vi "PathVelocityProfile.vi"(0 "Pose":dbl[](array[numeric]), 1 "time":dbl, 3 "intervalo":dbl=0.016, 5 "estimatives":T2, 9 "Path  Smooth":dbl[][](array[numeric]), 11 "V_max":dbl format="%#_13g", 13 "Accel":dbl=10.0, 14 "DesAccel":dbl=15.0) -> (4 "Time X":dbl[](array[numeric]), 6 "Velocities X":dbl[](array[numeric]), 8 "Time Y":dbl[](array[numeric]), 10 "Velocities Y":dbl[](array[numeric]))   [LabVIEW 2023]
uses:
  Controle/VelocityProfileState.ctl
  <vilib>/Analysis/_algsub.llb/Real Vector Norm.vi
  <vilib>/Analysis/coordinate.llb/Wrap Angle (scalar).vi
  <vilib>/Analysis/NI_AAL_Angle.lvlib
  <vilib>/Analysis/NI_AALPro.lvlib
panel:
  in  "est_vy":dbl
  in  "est_vx":dbl
  out "VelocityProfile Y":T1[](array[typedef])
  out "VelocityProfile X":T1[](array[typedef])
  out "Velocity Profile Y":cluster{dbl[], dbl[]}[](graph)
  out "Velocity Profile X":cluster{dbl[], dbl[]}[](graph)
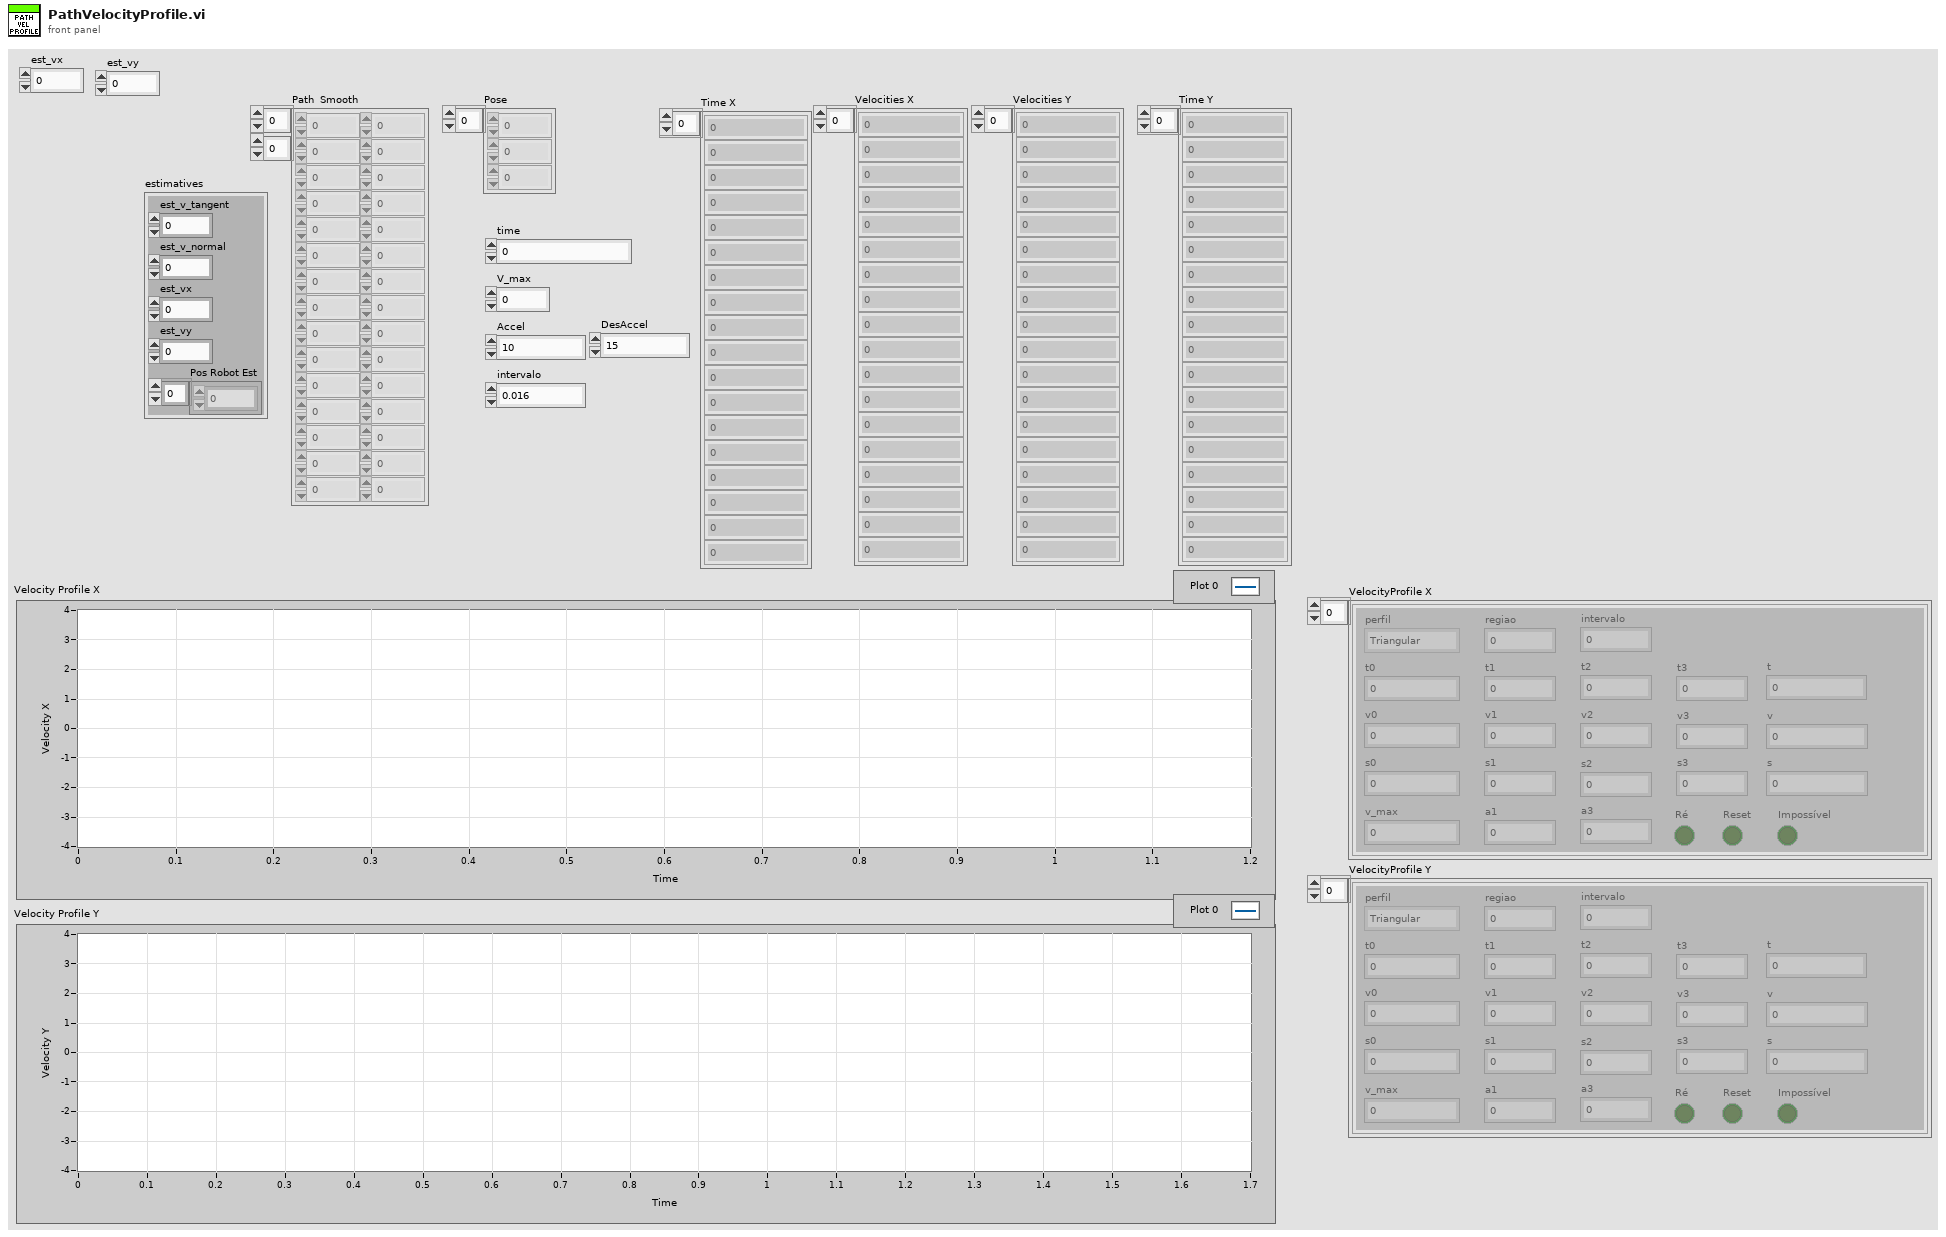
[diagram p1: front panel]
types:
  T1 = typedef "VelocityProfileState.ctl" = cluster{"t0":dbl, "t1":dbl, "t2":dbl, "t3":dbl, "v0":dbl, "v_max":dbl, "v3":dbl, "v2":dbl, "v1":dbl, "perfil":enum16{"Triangular", "Trapezoidal"}, "regiao":i32, "s0":dbl, "s1":dbl, "s2":dbl, "v":dbl, "t":dbl, "a1":dbl, "s3":dbl, "Reset":bool, "s":dbl, "a3":dbl, "Ré":bool, "Impossível":bool, "intervalo":dbl}
  T2 = cluster{"est_v_tangent":dbl, "est_v_normal":dbl, "est_vx":dbl, "est_vy":dbl, "Pos Robot Est":dbl[]}
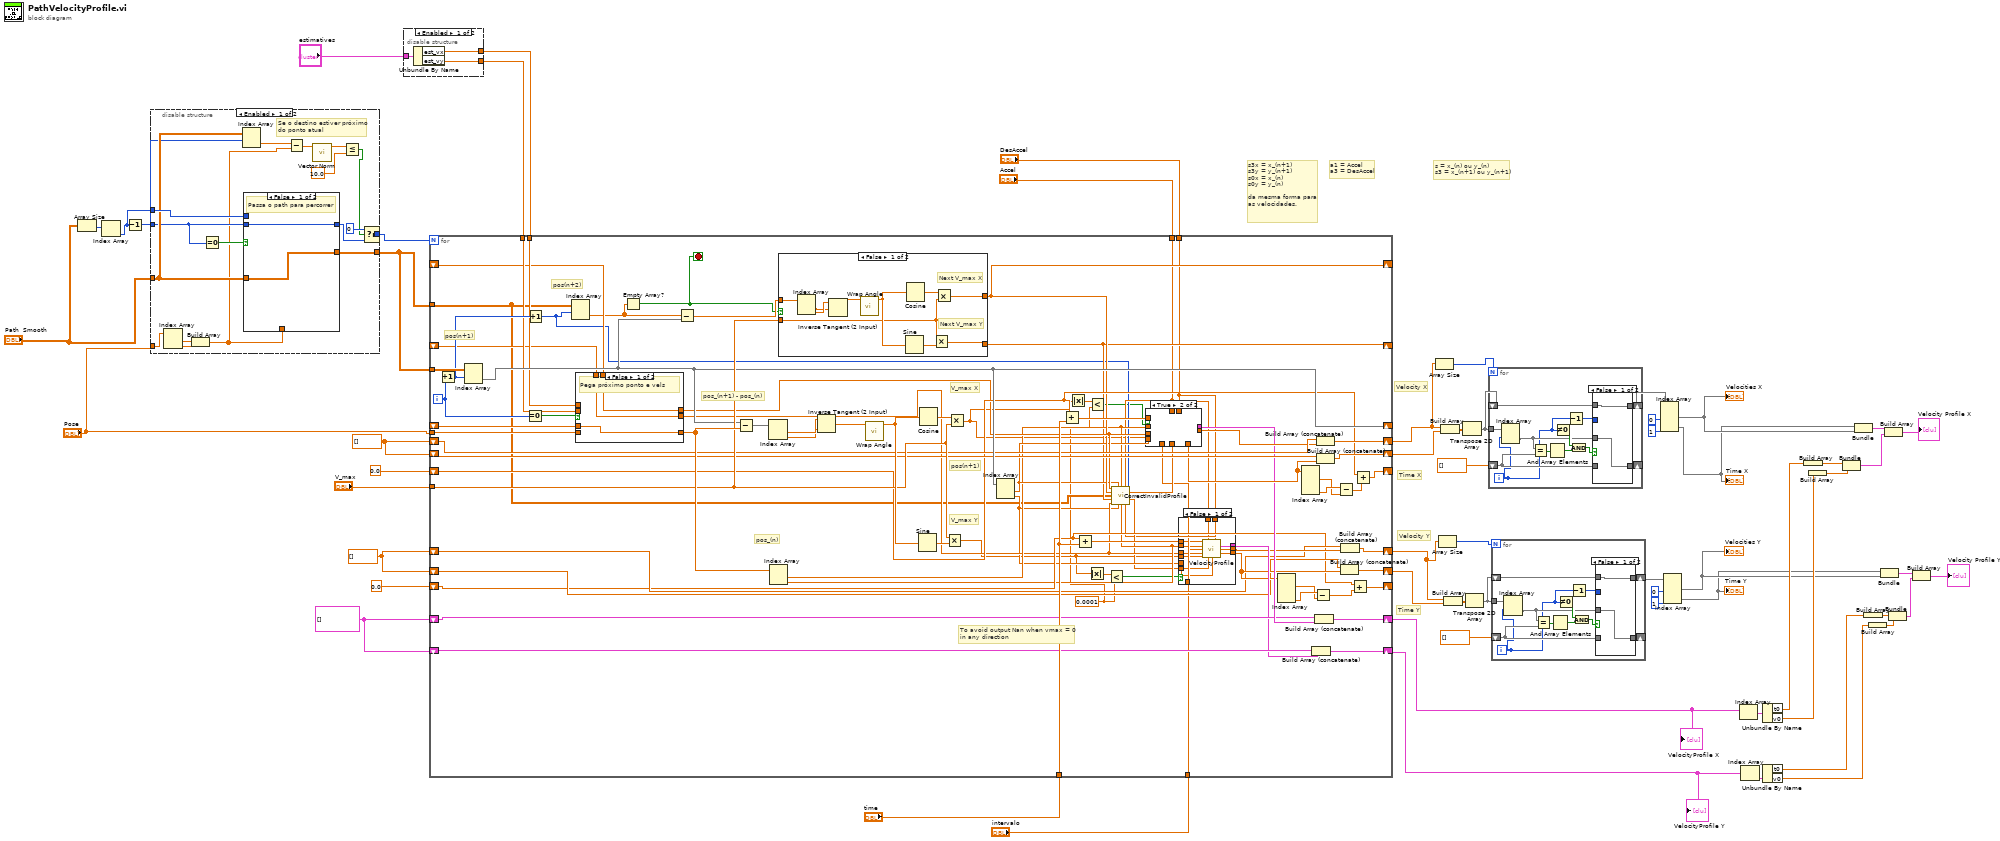
[diagram p0: block diagram]
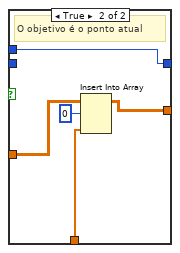
[diagram p2: hidden frame]
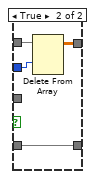
[diagram p4: hidden frame]
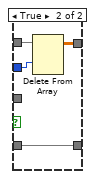
[diagram p5: hidden frame]
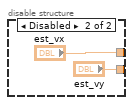
[diagram p6: hidden frame]
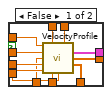
[diagram p7: hidden frame]
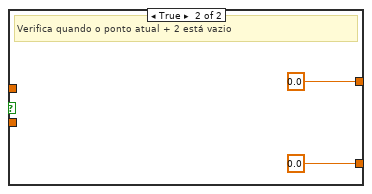
[diagram p9: hidden frame]
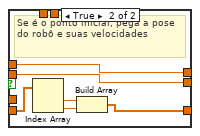
[diagram p10: hidden frame]
diagram:
  w48 = T1[] []
  w50 = dbl[] []
  w49 = dbl[] []
  # "s = x_(n) ou y_(n)\ns3 = x_(n+1) ou y_(n+1)"
  # "a1 = Accel\na3 = DesAccel"
  # "s3x = x_(n+1)\ns3y = y_(n+1)\ns0x = x_(n)\ns0y = y_(n)\n\nda mesma forma para\nas velocidades."
  # "Time X"
  # "Time Y"
  # "Velocity Y"
  # "Velocity X"
  n1 = Array Size(array="Path  Smooth") -> (size(s)=w53:i32[])
  n2 = Index Array(array=w53) -> (element=w6:i32)  [unwired: 1 in]
  n3 = Decrement(x=w6) -> (x-1=w3:i32)
  n4 = disable-structure shown="Enabled" {
    disable-tunnel: [w77 w85] -> w2
    disable-tunnel: w6 -> [w75 _]
    disable-tunnel: "Pose" -> [w74 _]
    disable-tunnel: [w71 w86] -> w1
    disable-tunnel: "Path  Smooth" -> [w68 w85]
    disable-tunnel: w3 -> [w67 w86]
    frame Enabled {
      # "Se o destino estiver próximo\ndo ponto atual"
      n5 = Index Array(array=w74) -> (element #1=w73:dbl, element #2=w72:dbl)  [unwired: 2 in]
      n6 = Build Array(w73, w72) -> (w65:dbl[])
      n7 = Equal To 0?(x=w67) -> (x = 0?=w76:bool)
      n8 = Index Array(array=w68, index (row)=w67) -> (element=w66:dbl[])  [unwired: 1 in]
      n9 = case shown="False" w76 {
        tunnel: [w78 w80] -> w77
        tunnel: w68 -> [w78 w82]
        tunnel: [w79 w84] -> w70
        tunnel: w67 -> [w79 _]
        tunnel: w75 -> [_ w84]
        tunnel: w65 -> [_ w83]
        frame False {
          # "Passa o path para percorrer"
        }
        frame True {
          # "O objetivo é o ponto atual"
          n10 = Insert Into Array(array=w82, index (row)=0, new element=w83) -> (w80:dbl[][])  [unwired: 1 in]
        }
      }
      n11 = Subtract(x=w66, y=w65) -> (x-y=w64:dbl[])
      n12 = call-poly <vilib>:"Vector Norm.vi"("Input Vector"=w64) -> ("norm"=w63:dbl)  [unwired: 9 in, 1 out]
      n13 = Less Or Equal?(x=w63, y=10.0) -> (x <= y?=w61:bool)
      n14 = Select(t=0, s=w61, f=w70) -> (s? t:f=w71:i32)
    }
    frame Disabled {
    }
  }
  n15 = disable-structure shown="Enabled" {
    disable-tunnel: "estimatives" -> [w89 _]
    disable-tunnel: [w88 "est_vx"] -> w52
    disable-tunnel: [w87 "est_vy"] -> w51
    frame Enabled {
      n16 = Unbundle By Name(w89) -> ("est_vx"=w88:dbl, "est_vy"=w87:dbl)
    }
    frame Disabled {
    }
  }
  n17 = for {
    N: w1 -> [_]
    tunnel: w2 -> [w150]
    tunnel: "Pose" -> [w166]
    shift-right: [w151] -> _
    shift-left: _ -> [w165]
    tunnel: "V_max" -> [w155]
    tunnel: "Accel" -> [w105]
    tunnel: "DesAccel" -> [w104]
    tunnel: w2 -> [w101]
    shift-right: [w119] -> _
    shift-left: 0.0 ("t3") -> [w121]
    shift-right: [w117] -> _
    shift-left: 0.0 ("t3") -> [w116]
    tunnel: "time" -> [w153]
    shift-right: [w144] -> w27
    shift-left: w49 -> [w149]
    shift-right: [w147] -> w30
    shift-left: w49 -> [w148]
    shift-right: [w125] -> w9
    shift-left: w50 -> [w123]
    shift-right: [w124] -> w10
    shift-left: w50 -> [w122]
    tunnel: w52 -> [w141]
    tunnel: w51 -> [w140]
    shift-right: [w114] -> _
    shift-left: _ -> [w139]
    shift-right: [w108] -> _
    shift-left: _ -> [w138]
    shift-right: [w130] -> w46
    shift-left: w48 -> [w133]
    shift-right: [w129] -> w45
    shift-left: w48 -> [w132]
    tunnel: "intervalo" -> [w99]
    i -> [w102]
    stop <- w142 stop-if-true
    w93 = 0.0001 ("y")
    # "To avoid output Nan when vmax = 0\nin any direction"
    # "pos(n+2)"
    # "pos(n+1)"
    # "pos(n+1)"
    # "pos_(n)"
    # "pos_(n+1) - pos_(n)"
    # "V_max Y"
    # "V_max X"
    n18 = Increment(x=w102) -> (x+1=w146:i32)
    n19 = Index Array(array=w150, index (row)=w146) -> (element=w151:dbl[])  [unwired: 1 in]
    n20 = Equal To 0?(x=w102) -> (x = 0?=w167:bool)
    n21 = Increment(x=w146) -> (x+1=w100:i32)
    n22 = Index Array(array=w101, index (row)=w100) -> (element=w103:dbl[])  [unwired: 1 in]
    n23 = case shown="False" w167 {
      tunnel: w166 -> [_ w212]
      tunnel: [w206 w209] -> w157
      tunnel: w165 -> [w206 _]
      tunnel: w141 -> [_ w208]
      tunnel: w140 -> [_ w207]
      tunnel: [w204 w208] -> w115
      tunnel: [w205 w207] -> w110
      tunnel: w139 -> [w204 _]
      tunnel: w138 -> [w205 _]
      frame False {
        # "Pega próximo ponto e vels"
      }
      frame True {
        # "Se é o ponto inicial, pega a pose\ndo robô e suas velocidades"
        n24 = Index Array(array=w212) -> (element #1=w211:dbl, element #2=w210:dbl)  [unwired: 2 in]
        n25 = Build Array(w211, w210) -> (w209:dbl[])
      }
    }
    n26 = Empty Array?(array=w103) -> (empty?=w142:bool)
    n27 = Subtract(x=w103, y=w151) -> (x-y=w156:dbl[])
    n28 = Subtract(x=w151, y=w157) -> (x-y=w163:dbl[])
    n29 = Index Array(array=w163) -> (element #1=w164:dbl, element #2=w162:dbl)  [unwired: 2 in]
    n30 = Index Array(array=w157) -> (element #1=w112:dbl, element #2=w111:dbl)  [unwired: 2 in]
    n31 = case shown="False" w142 {
      tunnel: w156 -> [w196 _]
      tunnel: w155 -> [w194 _]
      tunnel: [w193 0.0] -> w114
      tunnel: [w192 0.0] -> w108
      frame False {
        # "Next V_max Y"
        # "Next V_max X"
        n32 = Index Array(array=w196) -> (element #1=w195:dbl, element #2=w197:dbl)  [unwired: 2 in]
        n33 = Inverse Tangent (2 Input)(1:w195, 2:w197) -> (0:w198:dbl)
        n34 = call-poly <vilib>:"Wrap Angle.vi"("angle in"=w198) -> ("angle out"=w199:dbl)  [unwired: 9 in, 1 out]
        n35 = Sine(x=w199) -> (sin(x)=w201:dbl)
        n36 = Cosine(x=w199) -> (cos(x)=w200:dbl)
        n37 = Multiply(x=w194, y=w201) -> (x*y=w192:dbl)
        n38 = Multiply(x=w200, y=w194) -> (x*y=w193:dbl)
      }
      frame True {
        # "Verifica quando o ponto atual + 2 está vazio"
      }
    }
    n39 = Inverse Tangent (2 Input)(1:w164, 2:w162) -> (0:w161:dbl)
    n40 = call-poly <vilib>:"Wrap Angle.vi"("angle in"=w161) -> ("angle out"=w160:dbl)  [unwired: 9 in, 1 out]
    n41 = Sine(x=w160) -> (sin(x)=w158:dbl)
    n42 = Cosine(x=w160) -> (cos(x)=w159:dbl)
    n43 = Multiply(x=w155, y=w158) -> (x*y=w98:dbl)
    n44 = Multiply(x=w159, y=w155) -> (x*y=w94:dbl)
    n45 = Index Array(array=w151) -> (element #1=w113:dbl, element #2=w109:dbl)  [unwired: 2 in]
    n46 = Add(x=w121, y=w153) -> (x+y=w154:dbl)
    n47 = Absolute Value(x=w94) -> (abs(x)=w95:dbl)
    n48 = Add(x=w116, y=w153) -> (x+y=w152:dbl)
    n49 = Absolute Value(x=w98) -> (abs(x)=w97:dbl)
    n50 = Less?(x=w95, y=w93) -> (x < y?=w92:bool)
    n51 = Less?(x=w97, y=w93) -> (x < y?=w96:bool)
    n52 = call "CorrectInvalidProfile.vi"("v0x"=w115, "s3x"=w113, "s0x"=w112, "a1"=w105, "index"=w100, "v3x"=w114, "Path  Smooth"=w101, "v3y"=w108, "v0y"=w110, "s3y"=w109, "s0y"=w111, "a3"=w104) -> ("New v3x"=w106:dbl, "New v3y"=w107:dbl)  [unwired: 2 in]
    n53 = case shown="True" w92 {
      tunnel: w94 -> [w179 _]
      tunnel: w154 -> [w178 _]
      tunnel: [w177 _] -> w145
      tunnel: [w176 _] -> w143
      tunnel: [w175 _] -> w134
      tunnel: w115 -> [w174 _]
      tunnel: w113 -> [w173 _]
      tunnel: w112 -> [w172 _]
      tunnel: w106 -> [w171 _]
      tunnel: w105 -> [w170 _]
      tunnel: w104 -> [w169 _]
      tunnel: w99 -> [w168 _]
      frame False {
        n54 = call "VelocityProfile.vi"("t"=w178, "a1"=w170, "a3"=w169, "s"=w172, "intervalo"=w168, "v_est"=w174, "v_max"=w179, "v3"=w171, "s3"=w173) -> ("VelocityProfileState Out"=w175:T1, "Velocities"=w177:dbl[], "Time"=w176:dbl[])  [unwired: 3 in, 1 out]
      }
      frame True {
      }
    }
    n55 = case shown="False" w96 {
      tunnel: w98 -> [w191 _]
      tunnel: w152 -> [w190 _]
      tunnel: [w189 _] -> w131
      tunnel: [w188 _] -> w128
      tunnel: [w187 _] -> w126
      tunnel: w111 -> [w186 _]
      tunnel: w110 -> [w185 _]
      tunnel: w109 -> [w184 _]
      tunnel: w107 -> [w183 _]
      tunnel: w105 -> [w182 _]
      tunnel: w104 -> [w181 _]
      tunnel: w99 -> [w180 _]
      frame False {
        n56 = call "VelocityProfile.vi"("t"=w190, "a1"=w182, "a3"=w181, "s"=w186, "intervalo"=w180, "v_est"=w185, "v_max"=w191, "v3"=w183, "s3"=w184) -> ("VelocityProfileState Out"=w189:T1, "Velocities"=w188:dbl[], "Time"=w187:dbl[])  [unwired: 3 in, 1 out]
      }
      frame True {
      }
    }
    n57 = Index Array(array=w126) -> (element #1=w136:dbl, element #4=w137:dbl)  [unwired: 4 in, 2 out]
    n58 = Index Array(array=w143) -> (element #1=w127:dbl, element #4=w135:dbl)  [unwired: 4 in, 2 out]
    n59 = Build Array (concatenate)(w132, w131) -> (w129:T1[])
    n60 = Subtract(x=w137, y=w136) -> (x-y=w118:dbl)
    n61 = Build Array (concatenate)(w133, w134) -> (w130:T1[])
    n62 = Build Array (concatenate)(w149, w145) -> (w144:dbl[])
    n63 = Build Array (concatenate)(w148, w143) -> (w147:dbl[])
    n64 = Subtract(x=w135, y=w127) -> (x-y=w120:dbl)
    n65 = Build Array (concatenate)(w122, w126) -> (w124:dbl[])
    n66 = Build Array (concatenate)(w123, w128) -> (w125:dbl[])
    n67 = Add(x=w116, y=w118) -> (x+y=w117:dbl)
    n68 = Add(x=w121, y=w120) -> (x+y=w119:dbl)
  }
  "VelocityProfile X" <- w46
  "VelocityProfile Y" <- w45
  n69 = Array Size(array=w27) -> (size(s)=w24:i32)
  n70 = Array Size(array=w9) -> (size(s)=w13:i32)
  n71 = Build Array(w27, w30) -> (w23:dbl[][])
  n72 = Build Array(w9, w10) -> (w14:dbl[][])
  n73 = Transpose 2D Array(2D array=w23) -> (transposed array=w22:dbl[][])
  n74 = Transpose 2D Array(2D array=w14) -> (transposed array=w15:dbl[][])
  n75 = for {
    N: w24 -> [_]
    tunnel: w22 -> [w216]
    shift-right: [w224] -> _
    shift-left: dbl[] [] -> [w223]
    shift-right: [w217] -> w25
    shift-left: w22 -> [w218]
    i -> [w213]
    n76 = Index Array(array=w216, index (row)=w213) -> (element=w215:dbl[])  [unwired: 1 in]
    n77 = Equal?(x=w215, y=w223) -> (x = y?=w222:bool[])
    n78 = And Array Elements(Boolean array=w222) -> (logical AND=w221:bool)
    n79 = Not Equal To 0?(x=w213) -> (x != 0?=w220:bool)
    n80 = Decrement(x=w213) -> (x-1=w214:i32)
    n81 = And(x=w220, y=w221) -> (x .and. y?=w219:bool)
    n82 = case shown="False" w219 {
      tunnel: w215 -> [w226 _]
      tunnel: [w226 w230] -> w224
      tunnel: w223 -> [_ w230]
      tunnel: w218 -> [w225 w229]
      tunnel: [w225 w228] -> w217
      tunnel: w214 -> [_ w227]
      frame False {
      }
      frame True {
        n83 = Delete From Array(array=w229, index (row)=w227) -> (array with subset deleted=w228:dbl[][])  [unwired: 2 in, 1 out]
      }
    }
  }
  n84 = for {
    N: w13 -> [_]
    tunnel: w15 -> [w234]
    shift-right: [w242] -> _
    shift-left: dbl[] [] -> [w241]
    shift-right: [w235] -> w12
    shift-left: w15 -> [w236]
    i -> [w231]
    n85 = Index Array(array=w234, index (row)=w231) -> (element=w233:dbl[])  [unwired: 1 in]
    n86 = Equal?(x=w233, y=w241) -> (x = y?=w240:bool[])
    n87 = And Array Elements(Boolean array=w240) -> (logical AND=w239:bool)
    n88 = Not Equal To 0?(x=w231) -> (x != 0?=w238:bool)
    n89 = Decrement(x=w231) -> (x-1=w232:i32)
    n90 = And(x=w238, y=w239) -> (x .and. y?=w237:bool)
    n91 = case shown="False" w237 {
      tunnel: w233 -> [w244 _]
      tunnel: [w244 w248] -> w242
      tunnel: w241 -> [_ w248]
      tunnel: w236 -> [w243 w247]
      tunnel: [w243 w246] -> w235
      tunnel: w232 -> [_ w245]
      frame False {
      }
      frame True {
        n92 = Delete From Array(array=w247, index (row)=w245) -> (array with subset deleted=w246:dbl[][])  [unwired: 2 in, 1 out]
      }
    }
  }
  n93 = Index Array(array=w25, index (col) #1=0 ("disabled index (col)"), index (col) #2=1 ("index (col)")) -> (element #1=w29:dbl[], element #2=w28:dbl[])  [unwired: 2 in]
  "Velocities X" <- w29
  "Time X" <- w28
  n94 = Index Array(array=w12, index (col) #1=0 ("disabled index (col)"), index (col) #2=1 ("index (col)")) -> (element #1=w8:dbl[], element #2=w7:dbl[])  [unwired: 2 in]
  "Velocities Y" <- w8
  "Time Y" <- w7
  n95 = Index Array(array=w46) -> (element=w44:T1)  [unwired: 1 in]
  n96 = Index Array(array=w45) -> (element=w43:T1)  [unwired: 1 in]
  n97 = Unbundle By Name(w44) -> ("t0"=w36:dbl, "v0"=w35:dbl)
  n98 = Unbundle By Name(w43) -> ("t0"=w32:dbl, "v0"=w31:dbl)
  n99 = Build Array(w36) -> (w37:dbl[])
  n100 = Build Array(w35) -> (w38:dbl[])
  n101 = Bundle(w37, w38) -> (w18:cluster{dbl[], dbl[]})  [unwired: 1 in]
  n102 = Bundle(w28, w29) -> (w42:cluster{dbl[], dbl[]})  [unwired: 1 in]
  n103 = Build Array(w32) -> (w33:dbl[])
  n104 = Build Array(w31) -> (w34:dbl[])
  n105 = Bundle(w7, w8) -> (w40:cluster{dbl[], dbl[]})  [unwired: 1 in]
  n106 = Build Array(w42, w18) -> (→"Velocity Profile X":cluster{dbl[], dbl[]}[])
  n107 = Bundle(w33, w34) -> (w19:cluster{dbl[], dbl[]})  [unwired: 1 in]
  n108 = Build Array(w40, w19) -> (→"Velocity Profile Y":cluster{dbl[], dbl[]}[])
